vi "jsq_load.vi"(8 "error in (no error)":errorcluster, 11 "Open":path=path "C:/Users/Adam/Desktop/test.osq") -> (0 "error out":errorcluster, 2 "SEQs":T1[](array[typedef]), 3 "json file path(duplicate)":path, 4 "Lines":i32)   [LabVIEW 2015, in "oskar_tools.lvlib"]
uses:
  oskar_tools.lvlib
  seq_line.ctl
panel:
  out "json":string
  in  "Template":T1[](array[typedef])
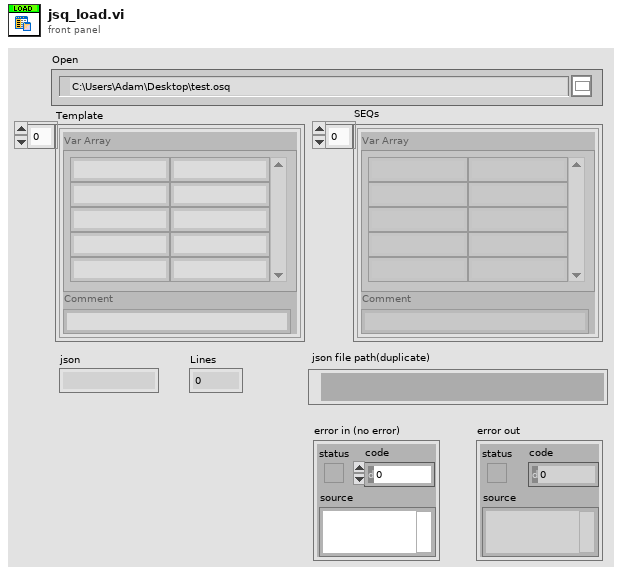
[diagram p1: front panel]
types:
  T1 = typedef "oskar_tools.lvlib/seq_line.ctl" = cluster{"Var Array":string[][], "Comment":string}
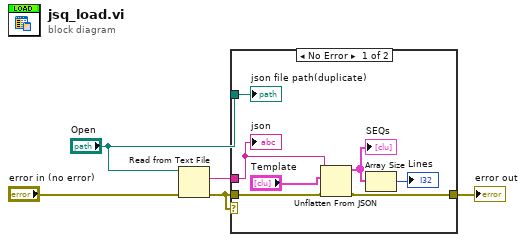
[diagram p0: block diagram]
diagram:
  n1 = Read from Text File(file (use dialog)="Open", error in="error in (no error)") -> (text=w2:string, error out=w3:errorcluster)  [unwired: 2 in, 2 out]
  n2 = case shown="No Error" w3 {
    tunnel: "Open" -> [w12 _]
    tunnel: w2 -> [w6 _]
    tunnel: w3 -> [w10 w13]
    tunnel: [w9 w13] -> w5
    frame No Error {
      n3 = Unflatten From JSON(JSON string=w6, type and defaults="Template", error in (no error)=w10) -> (value=w8:T1[], error out=w9:errorcluster)  [unwired: 4 in]
      "SEQs" <- w8
      n4 = Array Size(array=w8) -> (size(s)=→"Lines":i32)
      "json file path(duplicate)" <- w12
      "json" <- w6
    }
    frame Error {
    }
  }
  "error out" <- w5
